vi "Test Component A Does Something.vi"(11 "Test Case In":refnum<class "Component B Another Test.lvclass">) -> (0 "error out":errorcluster, 3 "Test Case Out":refnum<class "Component B Another Test.lvclass">)   [LabVIEW 2020, in "Component B Test Suite.lvlib" / "Component B Another Test.lvclass"]
uses:
  Component B Another Test.lvclass
  Component B Another Test.lvclass/Component B Another Test.ctl
  f6f40d18-eeda-474a-a6f8-b2449c055277.vi
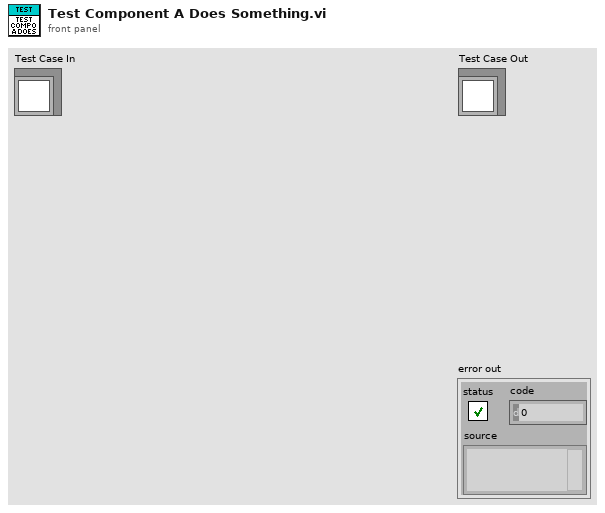
[diagram p1: front panel]
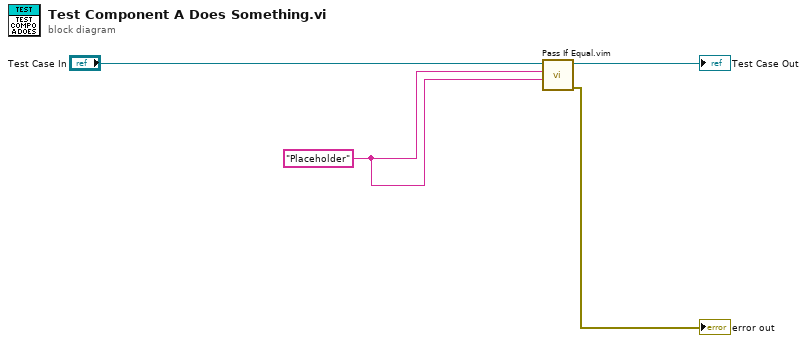
[diagram p0: block diagram]
diagram:
  w1 = "Placeholder"
  n1 = call "Pass If Equal.vim"("Actual"=w1, "Expected"=w1, "LUnit Test Case In"="Test Case In") -> ("error out"=→"error out":errorcluster, "LUnit Test Case Out"=→"Test Case Out":refnum<class "Component B Another Test.lvclass">)  [unwired: 7 in]
